vi "Main.vi"() -> ()   [LabVIEW 2024]
uses:
  <vilib>/Platform/TimedLoop/XDataNode/timing_clust.ctl
  <vilib>/Platform/TimedLoop/XDataNode/nitl_modes.ctl
  <vilib>/Platform/TimedLoop/XDataNode/wakeup.ctl
  <vilib>/addons/Maxon Motor/EPOS2 CANopen/CANopen/sbCANopenBaseClass.lvclass
  <vilib>/platform/TimedLoop/XDataNode/XDataNode.xnode
  <vilib>/Platform/TimedLoop/XDataNode/XDNodeRunTimeDep.lvlib
panel:
  out "ResetPID":bool
  in  "Motor_index":i32[](array[numeric])=[3, 6, 9, 12, 2, 7, 8, 13, 4, 5, 10, 11, 1, 14]
  out "canERROR":errorcluster[][](array[cluster])
  in  "Control Mode":string="O"
  in  "goal_Tensions":dbl[](array[numeric])
  in  "TARE":bool
  in  "curr_Tensions":dbl[](array[numeric])
  out "DAQ Error":errorcluster
  out "Write Late?":bool
  out "Write Time [us]":i64
  in  "Tare_Tensions":dbl[](array[numeric])=[1.6875269817998764, 0.7228096971601798, 1.962272927280566, 2.6696462364433735, 2.7003690389898463, 3.088938448864716, 1.6430905755314908, 3.0754139877790347, 3.5546581214666455, 3.2737863413382597, 4.727265898547672, 2.6001067118162604, 1.980007529135911, 1.8614502099489874]
  in  "STOP CONTROLLER":bool
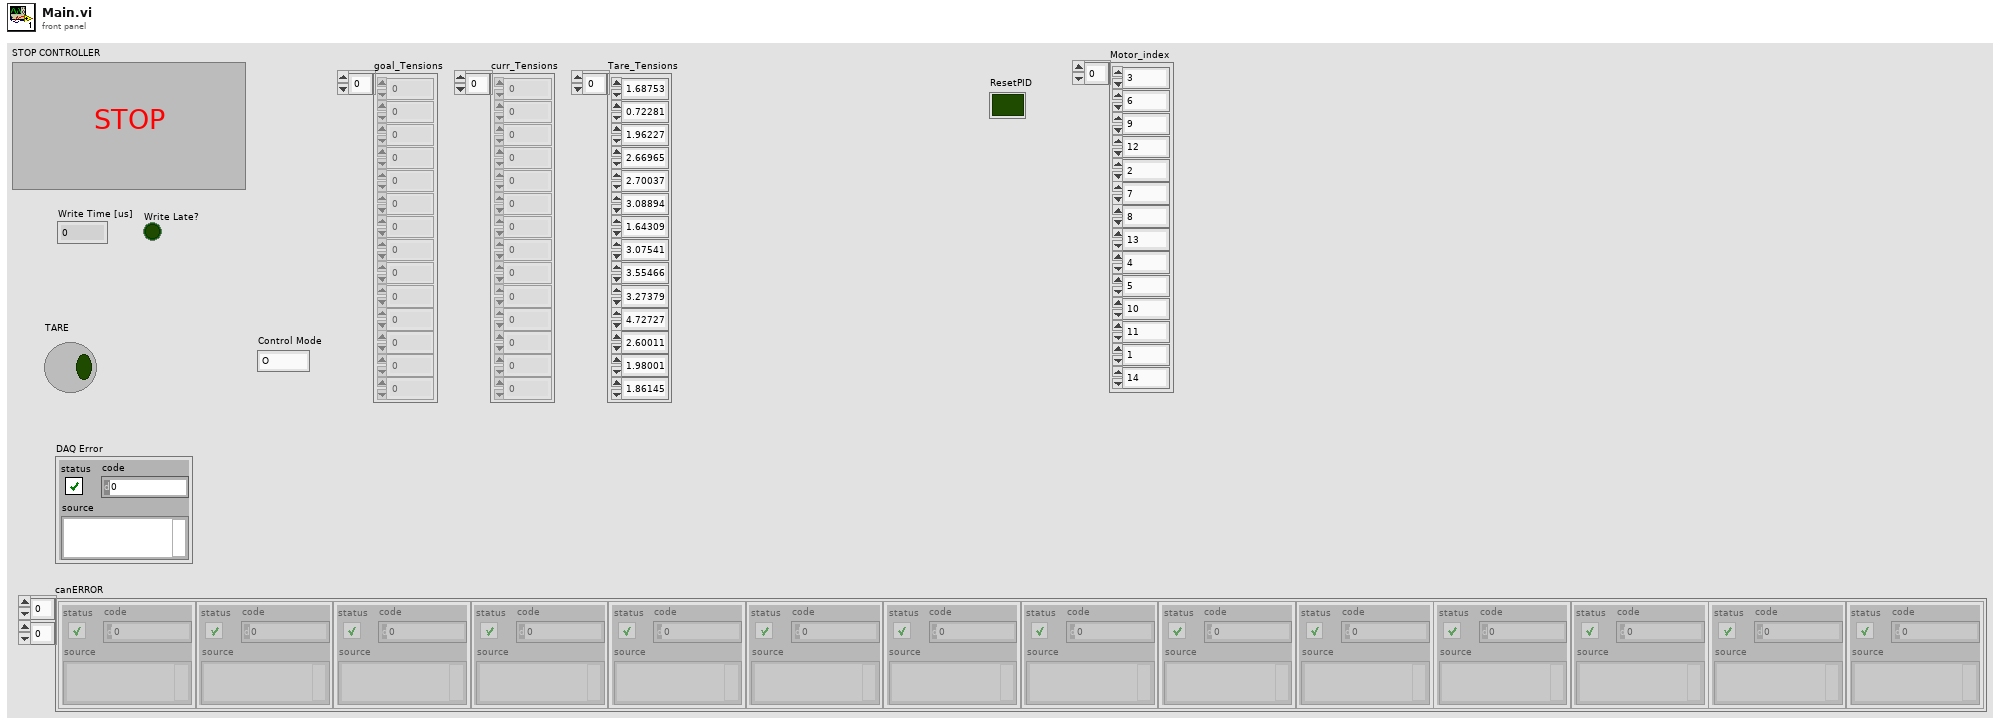
[diagram p1: front panel]
types:
  T1 = typedef "XDNodeRunTimeDep.lvlib/timing_clust.ctl" = cluster{"Expected End [f-1]":u64, "Actual End [f-1]":u64, "Finished Late? [f-1]":bool, "Expected End [i-1]":u64, "Actual End [i-1]":u64, "Finished Late? [i-1]":bool, "Expected Start [i]":u64, "Actual Start [i]":u64, "Expected Start [f]":u64, "Actual Start [f]":u64, "Source Name":string, "Structure Name":string, "Period":i64, "Deadline":i64, "Offset":i64, "Start":i64, "Priority":i32, "Timeout":i32, "Mode":T2, "Wakeup Reason":T3, "Error":errorcluster, "Source Type":string, "Secondary Source Type":string, "Global End Time":u64, "Global Start Time":u64, "Frame Duration":u64, "Iteration Duration":u64, "Assigned CPU":i32, "I/O Scan Engine Mode":u32}
  T2 = typedef "XDNodeRunTimeDep.lvlib/nitl_modes.ctl" = enum32{"No Change", "Process missed periods, maintain original phase", "Discard missed periods, maintain original phase", "Process missed periods, ignore original phase", "Discard missed periods, ignore original phase"}
  T3 = typedef "XDNodeRunTimeDep.lvlib/wakeup.ctl" = enum32{"Normal", "Aborted", "Asynchronous wakeup", "Timing source error", "Timed loop error", "Timeout"}
  T4 = cluster{"curr_Tensions":dbl[], "goal_Tensions":dbl[]}
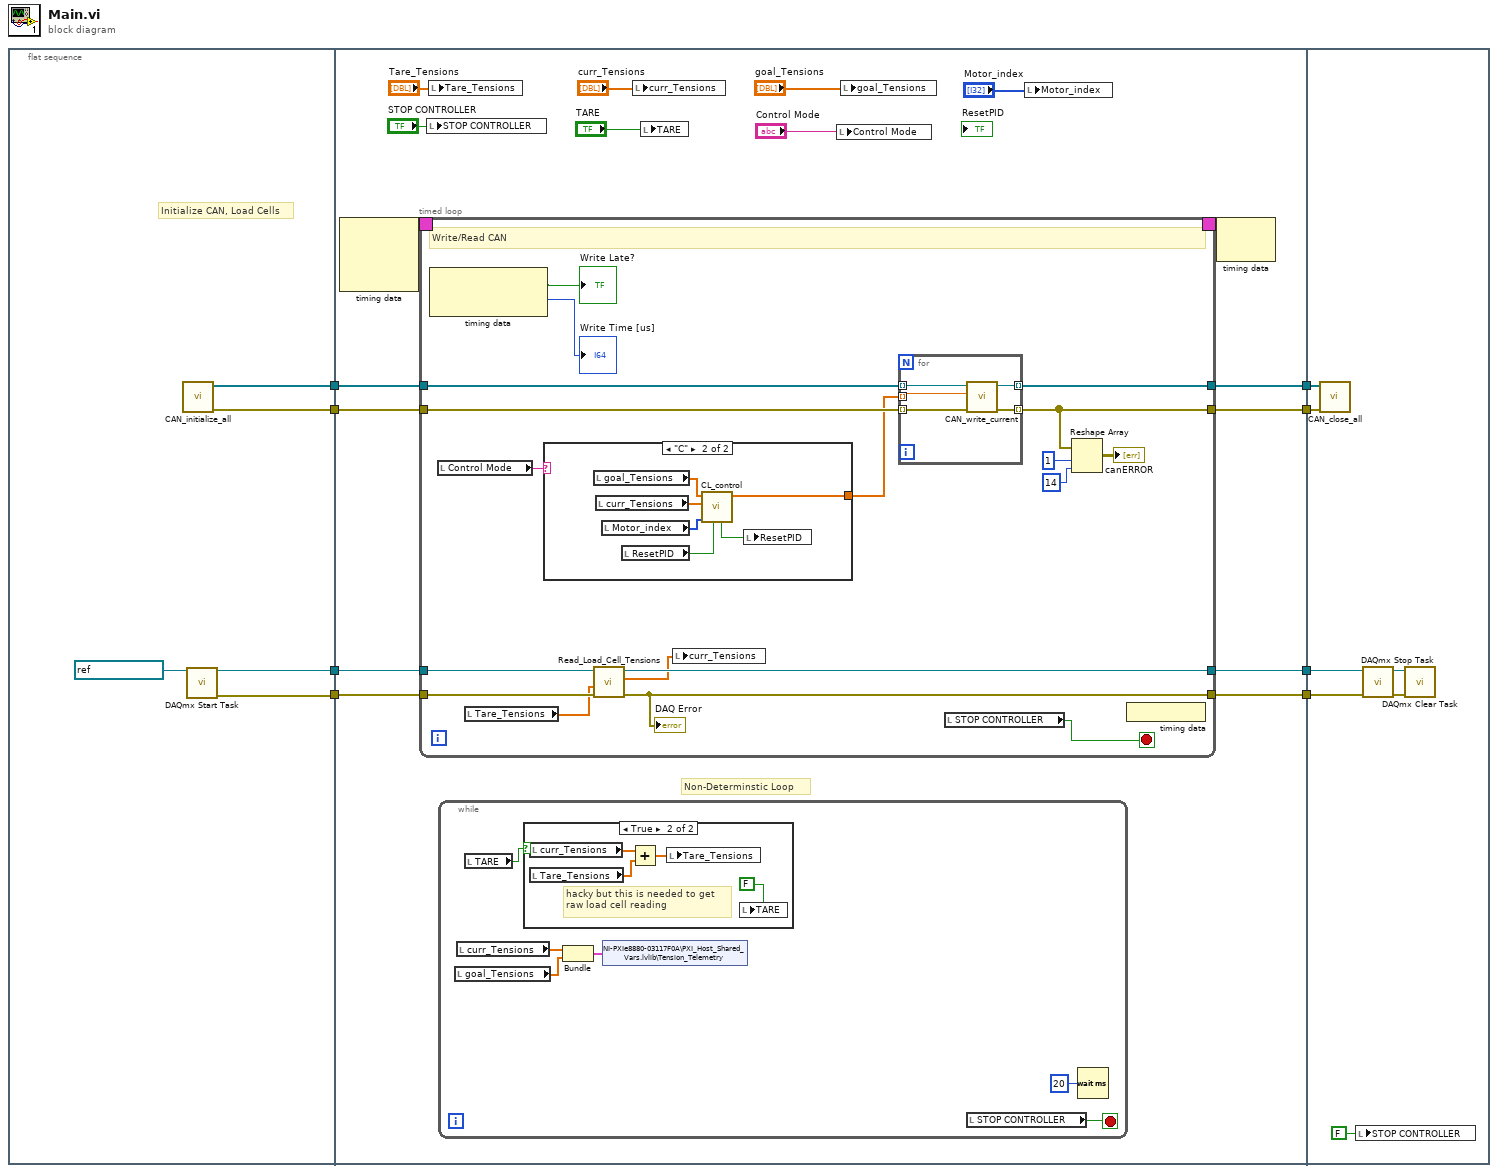
[diagram p0: block diagram]
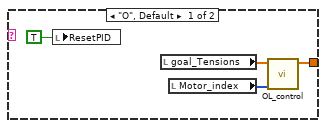
[diagram p3: hidden frame]
diagram:
  n1 = flat-sequence {
    tunnel: [w12] -> w8
    tunnel: [w13] -> w7
    tunnel: [w9] -> w4
    tunnel: [w10] -> w3
    tunnel: w8 -> [w28]
    tunnel: w7 -> [w27]
    tunnel: [w26] -> w6
    tunnel: [w25] -> w5
    tunnel: w4 -> [w23]
    tunnel: w3 -> [w22]
    tunnel: [w21] -> w2
    tunnel: [w20] -> w1
    tunnel: w6 -> [w86]
    tunnel: w5 -> [w85]
    tunnel: w2 -> [w82]
    tunnel: w1 -> [w81]
    frame #0 {
      # "Initialize CAN, Load Cells"
      n2 = call "CAN_initialize_all.vi"() -> ("Array of Canopen Sessions"=w13:refnum<class "sbCANopenBaseClass.lvclass">[], "Array of Error out's"=w12:errorcluster[])  [unwired: 5 in]
      n3 = call <vilib>:"DAQmx Start Task.vi"("task/channels in"=refnum<k21> "SCI_TenSen") -> ("task out"=w9:refnum<k21>, "error out"=w10:errorcluster)  [unwired: 13 in]
    }
    frame #1 {
      # "Non-Determinstic Loop"
      n4 = node-c288() -> (w30:T1)  [unwired: 3 in]
      n5 = timed-loop {
        tunnel: w28 -> [w50]
        tunnel: [w42] -> w26
        timing: w30 -> [_]
        timing-out: [_] -> w29
        tunnel: w27 -> [w51]
        tunnel: [w55] -> w25
        tunnel: w23 -> [w54]
        tunnel: w22 -> [w53]
        tunnel: [w52] -> w21
        tunnel: [w49] -> w20
        stop <- w56 stop-if-true
        # "Write/Read CAN"
        n6 = node-c288() -> (→"Write Late?":bool, →"Write Time [us]":i64)  [unwired: 1 in]
        n7 = local read "Control Mode"() -> (w47:string)
        n8 = local read "Tare_Tensions"() -> (w48:dbl[])
        n9 = case shown="\"C\"" w47 {
          tunnel: [w62 w68] -> w45
          frame "O", Default {
            n10 = local write "ResetPID"(TRUE) -> ()
            n11 = local read "goal_Tensions"() -> (w61:dbl[])
            n12 = local read "Motor_index"() -> (w60:i32[])
            n13 = call "OL_control.vi"("Motor_index"=w60, "goal_Tensions"=w61) -> ("can_Current"=w62:dbl[])  [unwired: 9 in]
          }
          frame "C" {
            n14 = local read "goal_Tensions"() -> (w67:dbl[])
            n15 = local read "curr_Tensions"() -> (w63:dbl[])
            n16 = local read "Motor_index"() -> (w66:i32[])
            n17 = local read "ResetPID"() -> (w65:bool)
            n18 = call "CL_control.vi"("ResetPID"=w65, "Motor_index"=w66, "curr_Tensions"=w63, "goal_Tensions"=w67) -> ("can_Current"=w68:dbl[], "Reset PID (output)"=w64:bool)  [unwired: 6 in]
            n19 = local write "ResetPID"(w64) -> ()
          }
        }
        n20 = call "Read_Load_Cell_Tensions.vi"("error in (no error)"=w53, "Tare Tension"=w48, "Refnum in"=w54) -> ("error out"=w49:errorcluster, "Measured Cable Tensions"=w46:dbl[], "Refnum out"=w52:refnum<k21>)  [unwired: 4 in]
        "DAQ Error" <- w49
        n21 = local write "curr_Tensions"(w46) -> ()
        n22 = for {
          tunnel: [w70] -> w55 mode=indexing
          tunnel: [w71] -> w42 mode=indexing
          tunnel: w51 -> [w73] mode=indexing
          tunnel: w50 -> [w72] mode=indexing
          tunnel: w45 -> [w69] mode=indexing
          n23 = call "CAN_write_current.vi"("error in"=w72, "Current Command [mA]"=w69, "CANopen Session In"=w73) -> ("error out"=w71:errorcluster, "CANopen Session Out"=w70:refnum<class "sbCANopenBaseClass.lvclass">)  [unwired: 7 in]
        }
        n24 = local read "STOP CONTROLLER"() -> (w56:bool)
        n25 = Reshape Array(w42, 1 ("dimension size"), 14 ("dimension size")) -> (→"canERROR":errorcluster[][])
        n26 = node-c288() -> ()  [unwired: 1 out]
      }
      n27 = local write "STOP CONTROLLER"("STOP CONTROLLER") -> ()
      n28 = local write "Tare_Tensions"("Tare_Tensions") -> ()
      n29 = while {
        stop <- w36 stop-if-true
        n30 = local read "goal_Tensions"() -> (w33:dbl[])
        n31 = local read "curr_Tensions"() -> (w34:dbl[])
        n32 = local read "TARE"() -> (w35:bool)
        n33 = case shown="True" w35 {
          frame False {
          }
          frame True {
            # "hacky but this is needed to get \nraw load cell reading"
            n34 = local read "curr_Tensions"() -> (w39:dbl[])
            n35 = local read "Tare_Tensions"() -> (w38:dbl[])
            n36 = Add(x=w39, y=w38) -> (x+y=w40:dbl[])
            n37 = local write "Tare_Tensions"(w40) -> ()
            n38 = local write "TARE"(FALSE ("TARE")) -> ()
          }
        }
        n39 = Bundle("curr_Tensions"=w34, "goal_Tensions"=w33) -> (w32:T4)  [unwired: 1 in]
        n40 = shared-variable "NI-PXIe8880-03117F0A\\PXI_Host_Shared_Vars.lvlib\\Tension_Telemetry"(w32) -> ()  [unwired: 1 in, 1 out]
        n41 = local read "STOP CONTROLLER"() -> (w36:bool)
        n42 = Wait (ms)(milliseconds to wait=u32 20) -> ()  [unwired: 1 out]
      }
      n43 = local write "curr_Tensions"("curr_Tensions") -> ()
      n44 = local write "TARE"("TARE") -> ()
      n45 = local write "Control Mode"("Control Mode") -> ()
      n46 = local write "goal_Tensions"("goal_Tensions") -> ()
      n47 = local write "Motor_index"("Motor_index") -> ()
      n48 = node-c288(w29) -> ()  [unwired: 1 out]
    }
    frame #2 {
      n49 = call "CAN_close_all.vi"("Input Error out array"=w86, "Input CANopen Sessions array"=w85) -> ()  [unwired: 10 in]
      n50 = local write "STOP CONTROLLER"(FALSE ("STOP CONTROLLER")) -> ()
      n51 = call <vilib>:"DAQmx Stop Task.vi"("task/channels in"=w82, "error in"=w81) -> ("task out"=w83:refnum<k21>, "error out"=w84:errorcluster)  [unwired: 12 in]
      n52 = call <vilib>:"DAQmx Clear Task.vi"("task in"=w83, "error in"=w84) -> ()  [unwired: 13 in, 1 out]
    }
  }
